vi "SetPolyIcon.vi"   [LabVIEW 2020]
types:
  T1 = cluster{"VIPath":path, "Menu Name":string, "Selector Name":string}[]
  T2 = typedef "imagedata.ctl" = cluster{"image type":i32, "image depth":i32, "image":u8[], "mask":u8[], "colors":u32[], "Rectangle":cluster{"left":i16, "top":i16, "right":i16, "bottom":i16}}
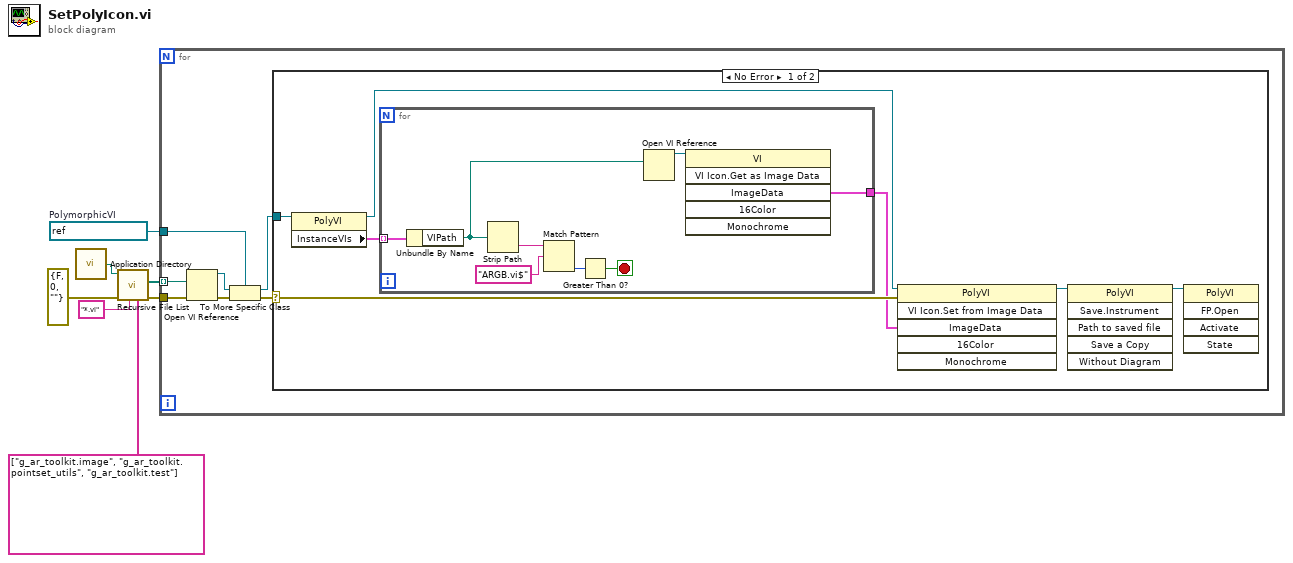
[diagram p0: block diagram]
diagram:
  w4 = refnum<vi> refnum  # PolymorphicVI
  n1 = call <vilib>:"Application Directory.vi"() -> ("Application Directory"=w3:path)
  n2 = call <vilib>:"Recursive File List.vi"("Folders to Exclude"=string[] ["g_ar_toolkit.image", "g_ar_toolkit.pointset_utils", "g_ar_toolkit.test"], "pattern"="*.vi", "error in (no error)"=errorcluster {"status"=FALSE, "code"=0, "source"=""} ("error out"), "Folder Path"=w3) -> ("error out"=w7:errorcluster, "All Files in Dir"=w6:path[])  [unwired: 3 in, 3 out]
  n3 = for {
    tunnel: w7 -> [w14]
    tunnel: w6 -> [w13] mode=indexing
    tunnel: w4 -> [w12]
    n4 = Open VI Reference(vi path=w13, error in (no error)=w14) -> (vi reference=w11:refnum<vi>, error out=w10:errorcluster)  [unwired: 4 in]
    n5 = To More Specific Class(target class=w12, reference=w11, error in=w10) -> (specific class reference=w8:refnum<vi>, error out=w9:errorcluster)
    n6 = case shown="No Error" w9 {
      selector: w9 -> [w21 _]
      tunnel: w8 -> [w20 _]
      frame No Error {
        n7 = property class="PolyVI"(reference=w20) -> (reference out=w19:refnum<vi>, "InstanceVIs"=w18:T1)  [unwired: 1 in, 1 out]
        n8 = for {
          tunnel: w18 -> [w29] mode=indexing
          tunnel: [w24] -> w17
          stop <- w23 stop-if-true
          n9 = Unbundle By Name(w29) -> ("VIPath"=w25:path)
          n10 = Strip Path(path=w25) -> (name=w28:string)  [unwired: 1 out]
          n11 = Match Pattern(string=w28, regular expression="ARGB.vi$") -> (offset past match=w26:i32)  [unwired: 1 in, 3 out]
          n12 = Greater Than 0?(x=w26) -> (x > 0?=w23:bool)
          n13 = Open VI Reference(vi path=w25) -> (vi reference=w22:refnum<vi>)  [unwired: 5 in, 1 out]
          n14 = invoke class="VI" method="VI Icon.Get as Image Data"(reference=w22) -> ("ImageData"=w24:T2)  [unwired: 5 in, 5 out]
        }
        n15 = invoke class="PolyVI" method="VI Icon.Set from Image Data"(reference=w19, error in=w21, "ImageData"=w17) -> (reference out=w16:refnum<vi>)  [unwired: 3 in, 5 out]
        n16 = invoke class="PolyVI" method="Save.Instrument"(reference=w16) -> (reference out=w15:refnum<vi>)  [unwired: 5 in, 5 out]
        n17 = invoke class="PolyVI" method="FP.Open"(reference=w15) -> ()  [unwired: 4 in, 5 out]
      }
      frame Error {
      }
    }
  }
